vi "subVI.vi"(8 "error in (no error)":errorcluster, 11 "Cluster in":T1) -> (3 "Cluster out":T1)   [LabVIEW 2014]
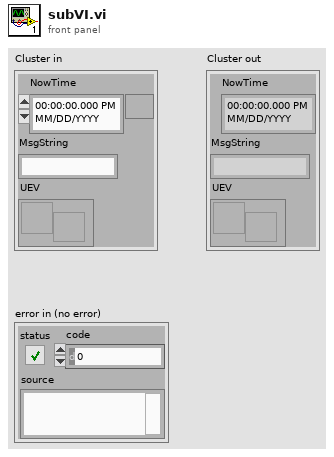
[diagram p1: front panel]
types:
  T1 = cluster{"NowTime":timestamp, "MsgString":string, "UEV":refnum<user-event>}
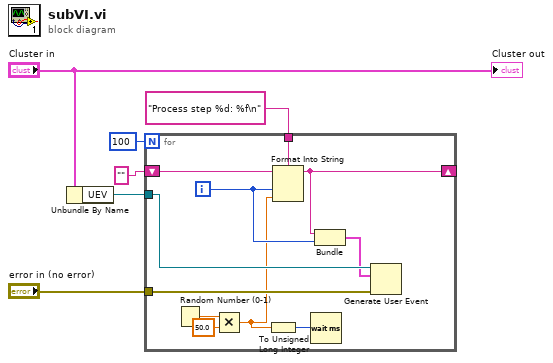
[diagram p0: block diagram]
diagram:
  n1 = Unbundle By Name("Cluster in") -> ("UEV"=w5:refnum<user-event>)
  n2 = for {
    N: 100 -> [_]
    tunnel: "error in (no error)" -> [w17]
    tunnel: w5 -> [w16]
    shift-right: [w10] -> _
    shift-left: "" -> [w15]
    tunnel: "Process step %d: %f\n" ("format string") -> [w8]
    i -> [w9]
    n3 = Random Number (0-1)() -> (number: 0 to 1=w14:dbl)
    n4 = Multiply(x=w14, y=50.0) -> (x*y=w7:dbl)
    n5 = To Unsigned Long Integer(number=w7) -> (unsigned 32bit integer=w12:u32)
    n6 = Format Into String(format string=w8, initial string=w15, w9, w7) -> (resulting string=w10:string)  [unwired: 1 in, 1 out]
    n7 = Wait (ms)(milliseconds to wait=w12) -> ()  [unwired: 1 out]
    n8 = Bundle(w10, w9) -> (w11:cluster{string, i32})  [unwired: 1 in]
    n9 = Generate User Event(user event=w16, event data cluster=w11, error in=w17) -> ()  [unwired: 1 in, 2 out]
  }
  "Cluster out" <- "Cluster in"
